vi "Dive_LDA_if_heater enabled off.vi"() -> ()   [LabVIEW 2022 SP3]
uses:
  Controls/User_Specific_mode.ctl
  Gen Trav/Trav_mode.ctl
panel:
  out "output array":sgl[](array[numeric])
  out "Heater Enable":bool
  in  "stop":bool
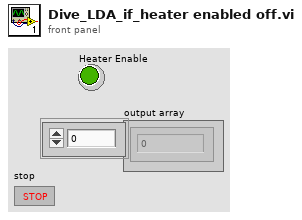
[diagram p1: front panel]
types:
  T1 = typedef "Trav_mode.ctl" = enum16{"Move traverse", "Read traverse position", "Teach Position"}
  T2 = typedef "User_Specific_mode.ctl" = enum16{"Check VI only", "Run VI"}
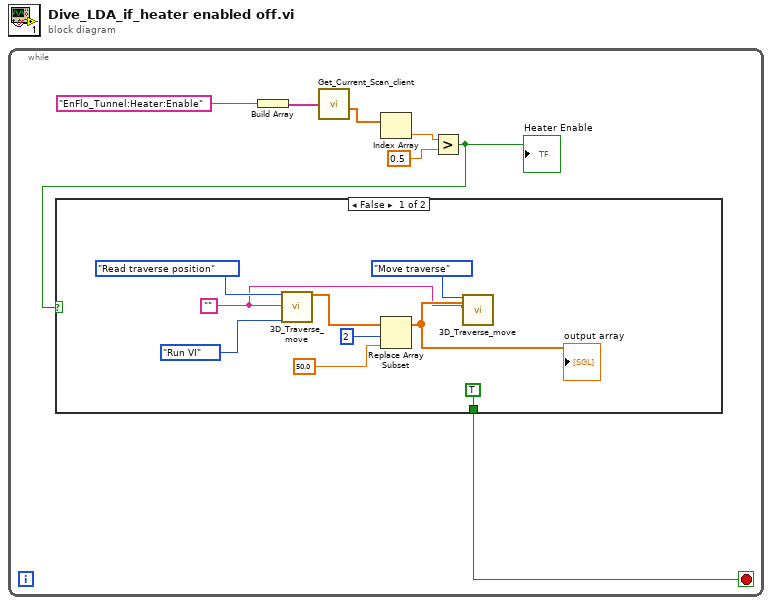
[diagram p0: block diagram]
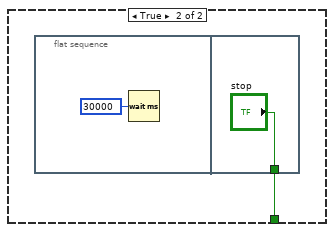
[diagram p2: hidden frame]
diagram:
  n1 = while {
    stop <- w1 stop-if-true
    n2 = Build Array("EnFlo_Tunnel:Heater:Enable") -> (w6:string[])
    n3 = call "Get_Current_Scan_client.vi"("ADAM Ch Names"=w6) -> ("Numerical Values"=w5:dbl[])  [unwired: 1 in, 2 out]
    n4 = Index Array(array=w5) -> (element=w4:dbl)  [unwired: 1 in]
    n5 = Greater?(x=w4, y=0.5) -> (0:w2:bool)
    "Heater Enable" <- w2
    n6 = case shown="False" w2 {
      tunnel: [TRUE ("stop") w17] -> w1
      frame False {
        w9 = ""
        n7 = call "3D_Traverse_move.vi"("Mode"=Trav_mode."Read traverse position", "Extra command String"=w9, "Simulate/Run"=User_Specific_mode."Run VI") -> ("Trav Position achieved"=w13:sgl[])  [unwired: 13 in, 3 out]
        n8 = Replace Array Subset(array=w13, new element=sgl 50.0 ("new element/subarray"), index=2) -> (w12:sgl[])
        "output array" <- w12
        n9 = call "3D_Traverse_move.vi"("Mode"=Trav_mode."Move traverse", "Position"=w12, "Extra command String"=w9) -> ()  [unwired: 13 in, 4 out]
      }
      frame True {
        n10 = flat-sequence {
          tunnel: ["stop"] -> w17
          frame #0 {
            n11 = Wait (ms)(milliseconds to wait=u32 30000) -> ()  [unwired: 1 out]
          }
          frame #1 {
          }
        }
      }
    }
  }
